vi "Equals.vi"(8 "error in (no error)":errorcluster, 10 "Data in":refnum<class "Data.lvclass">, 11 "String in":refnum<class "String.lvclass">) -> (0 "error out":errorcluster, 1 "Equals?":bool, 2 "Data out":refnum<class "Data.lvclass">, 3 "String out":refnum<class "String.lvclass">)   [LabVIEW 2015, in "MDSplus.lvlib" / "String.lvclass"]
uses:
  <vilib>/MDSplus/Classes/Data_Class/Scalar_Class/String_Class/String.lvclass
  <vilib>/MDSplus/Classes/Data_Class/Data.lvclass
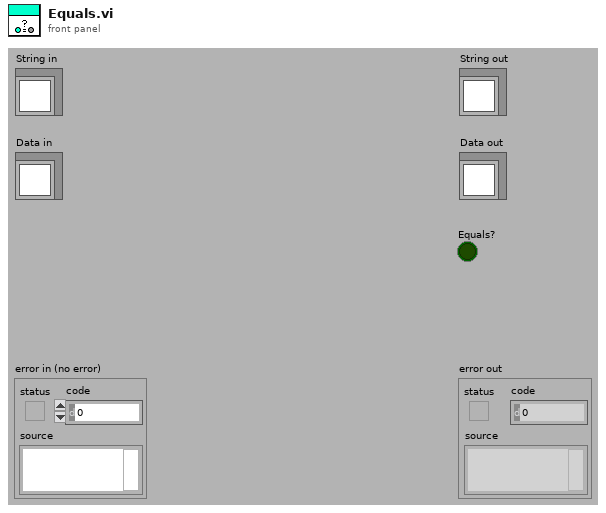
[diagram p1: front panel]
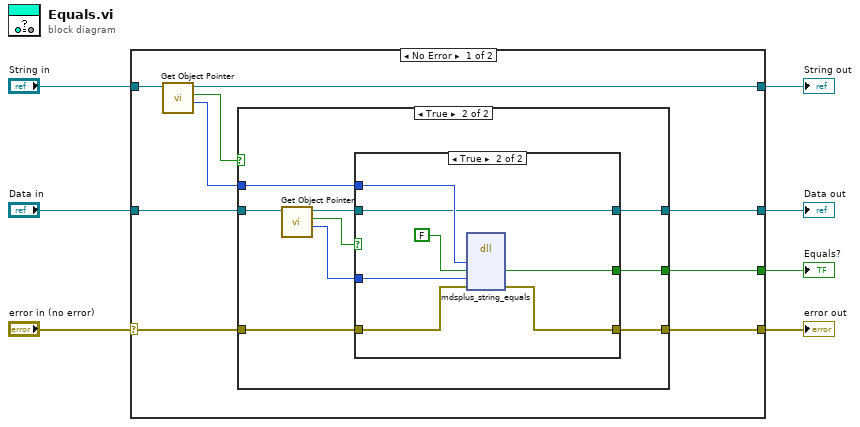
[diagram p0: block diagram]
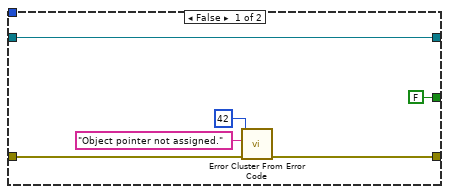
[diagram p2: hidden frame]
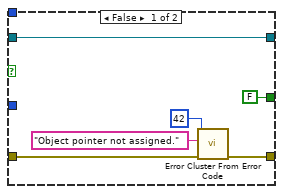
[diagram p3: hidden frame]
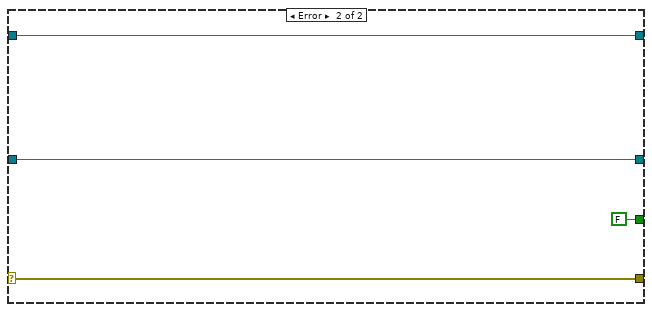
[diagram p4: hidden frame]
diagram:
  n1 = case shown="No Error" "error in (no error)" {
    selector: "error in (no error)" -> [w13 w48]
    tunnel: [w12 w48] -> w6
    tunnel: [w11 w47] -> w4
    tunnel: "String in" -> [w16 w47]
    tunnel: "Data in" -> [w10 w45]
    tunnel: [w9 w45] -> w2
    tunnel: [w8 FALSE] -> w1
    frame No Error {
      n2 = call-dynamic "Get Object Pointer.vi"("Data in"=w16) -> ("Object Pointer"=w14:i64, "Assigned object pointer?"=w15:bool, "Data out"=w11:refnum<class "String.lvclass">)  [unwired: 8 in]
      n3 = case shown="True" w15 {
        tunnel: w14 -> [_ w25]
        tunnel: w13 -> [w20 w31]
        tunnel: [w19 w30] -> w12
        tunnel: w10 -> [w18 w29]
        tunnel: [w18 w24] -> w9
        tunnel: [FALSE w23] -> w8
        frame False {
          n4 = call <vilib>:"Error Cluster From Error Code.vi"("error in (no error)"=w20, "error message (\"\")"="Object pointer not assigned." ("error message (\"\")"), "error code (0)"=42) -> ("error out"=w19:errorcluster)  [unwired: 6 in]
        }
        frame True {
          n5 = call-dynamic "Get Object Pointer.vi"("Data in"=w29) -> ("Object Pointer"=w26:i64, "Assigned object pointer?"=w27:bool, "Data out"=w28:refnum<class "Data.lvclass">)  [unwired: 8 in]
          n6 = case shown="True" w27 {
            tunnel: w31 -> [w34 w44]
            tunnel: [w33 w43] -> w30
            tunnel: w28 -> [w37 w40]
            tunnel: w26 -> [_ w41]
            tunnel: w25 -> [_ w42]
            tunnel: [w37 w40] -> w24
            tunnel: [FALSE w38] -> w23
            frame False {
              n7 = call <vilib>:"Error Cluster From Error Code.vi"("error in (no error)"=w34, "error message (\"\")"="Object pointer not assigned." ("error message (\"\")"), "error code (0)"=42) -> ("error out"=w33:errorcluster)  [unwired: 6 in]
            }
            frame True {
              n8 = dll-call lib="MDSobjectsLVShr" fn="mdsplus_string_equals"("lvStringPtr"=w42, "equalsOut"=FALSE, "lvDataPtrIn"=w41, "error"=w44) -> ("equalsOut"=w38:bool, "error"=w43:errorcluster)  [unwired: 6 in, 2 out]
            }
          }
        }
      }
    }
    frame Error {
    }
  }
  "error out" <- w6
  "String out" <- w4
  "Data out" <- w2
  "Equals?" <- w1
